vi "Keithley DMM6500 DAQ6500 Series Scanning Low Level DCV.vi"() -> ()   [LabVIEW 2016]
doc: "This example shows how to scan low level DC voltage."
uses:
  Public/Data/Read (Multiple Points).vi
  Keithley DMM6500 DAQ6500 Series.lvlib
panel:
  in  "Buffer Element2 ()":i32(ring) items=["", "Date", "Extra", "Formatted", "Fractional", "Reading", "Relative", "Seconds", "Status", "Time", "Tstamp", "Unit", "CHAN", "Extra Form", "Extra Unit"]
  in  "Buffer Element1 ()":i32(ring) items=["", "Date", "Extra", "Formatted", "Fractional", "Reading", "Relative", "Seconds", "Status", "Time", "Tstamp", "Unit", "CHAN", "Extra Format", "Extra Unit"]
  in  "File Name(\"/usb1/MyData.csv\")":string="/usb1/MyData.csv"
  out "Measurements":dbl[](array[numeric])
  in  "Scan Delay (0 s)":dbl
  in  "Power Line Cycle (1)":dbl=1.0
  in  "Scan Count (10)":u32=10
  in  "Buffer Size (10)":u32=10
  in  "Buffer Name(defbuffer1)":string="defbuffer1"
  in  "Channel List (\"101:106\")":string="101:106"
  in  "VISA resource name":refnum<visa-resource-name>
  # "(c) 2018 National Instruments.  ALL RIGHTS RESERVED."
  # "This example VI demonstrates how to use the DAQ6500 series to accurately measure DC voltage in a variety of ranges. To ensure accurate data, the NPLC (Number of Power Line Cycles) and autozero  options are used for this test."
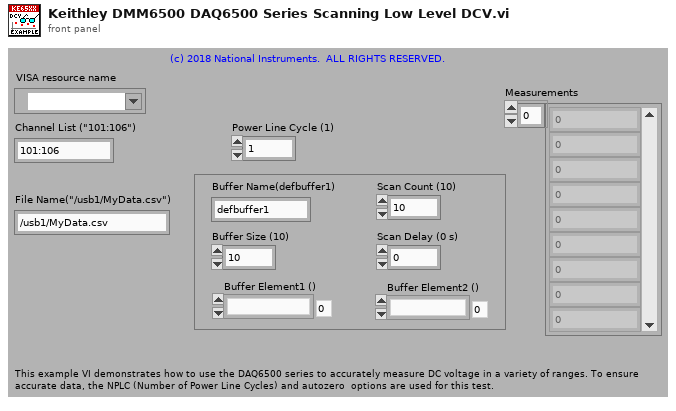
[diagram p1: front panel]
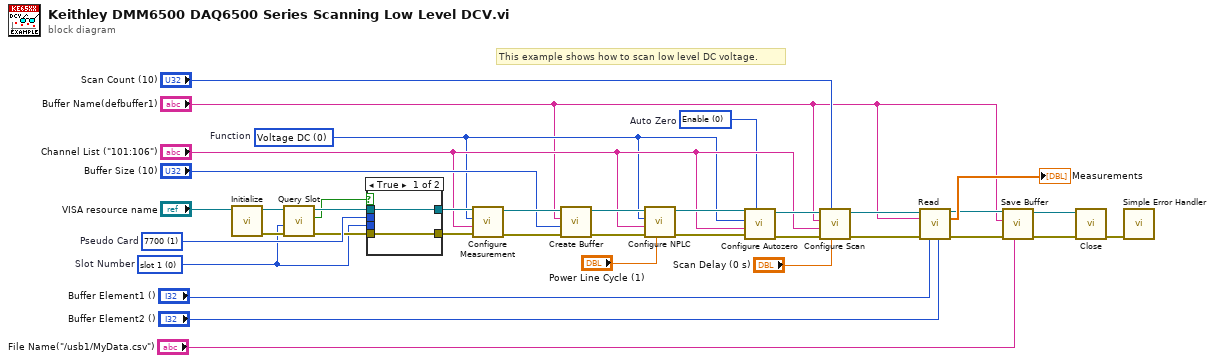
[diagram p0: block diagram]
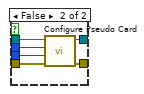
[diagram p2: hidden frame]
diagram:
  w4 = 0 items=["slot 1", "slot 2"]  # Slot Number
  w15 = 1 items=["0", "7700", "7701", "7702", "7703", "7705", "7706", "7707", "7708", "7709", "7710", "7711", "7712"]  # Pseudo Card
  w16 = u32 0 items=["Enable", "Disable", "Once"]  # Auto Zero
  w22 = 0 items=[" Voltage DC", "Voltage AC", "Current DC", "Current AC", "Resistance", "4-wire Resistance", "Diode", "Capacitance", "Temperature", "Continuity", "Frequency", "Period", "Voltage Ratio", "Digitize Voltage", "Digitize Current"]  # Function
  # "This example shows how to scan low level DC voltage."
  n1 = call "Initialize.vi"("VISA resource name"="VISA resource name") -> ("error out"=w7:errorcluster, "VISA resource name out"=w8:refnum<visa-resource-name>)  [unwired: 9 in]
  n2 = call "Query Slot.vi"("error in (no error)"=w7, "Slot Number(0: slot 1)"=w4, "VISA resource name"=w8) -> ("error out"=w6:errorcluster, "Real Card In Slot"=w3:bool, "VISA resource name out"=w5:refnum<visa-resource-name>)  [unwired: 6 in]
  n3 = case shown="True" w3 {
    tunnel: [w39 w45] -> w35
    tunnel: [w38 w44] -> w34
    tunnel: w15 -> [_ w43]
    tunnel: w6 -> [w38 w42]
    tunnel: w5 -> [w39 w41]
    tunnel: w4 -> [_ w40]
    frame True {
    }
    frame False {
      n4 = call "Configure Pseudo Card.vi"("error in (no error)"=w42, "Slot Number (0: slot1)"=w40, "Pseudo Card (0:No pseudocard)"=w43, "VISA resource name"=w41) -> ("error out"=w44:errorcluster, "VISA resource name out"=w45:refnum<visa-resource-name>)  [unwired: 6 in]
    }
  }
  n5 = call "Configure Measurement.vi"("error in (no error)"=w34, "Channel List(\"\")"="Channel List (\"101:106\")", "Function (0: Voltage DC)"=w22, "VISA resource name"=w35) -> ("error out"=w32:errorcluster, "VISA resource name out"=w33:refnum<visa-resource-name>)  [unwired: 6 in]
  n6 = call "Create Buffer.vi"("error in (no error)"=w32, "Buffer Size (10)"="Buffer Size (10)", "Buffer Name (\"\")"="Buffer Name(defbuffer1)", "VISA resource name"=w33) -> ("error out"=w29:errorcluster, "VISA resource name out"=w30:refnum<visa-resource-name>)  [unwired: 6 in]
  n7 = call "Configure NPLC.vi"("Power Line Cycle (1)"="Power Line Cycle (1)", "error in (no error)"=w29, "Channel List(\"\")"="Channel List (\"101:106\")", "Function (0: Voltage DC)"=w22, "VISA resource name"=w30) -> ("error out"=w27:errorcluster, "VISA resource name out"=w28:refnum<visa-resource-name>)  [unwired: 5 in]
  n8 = call "Configure Autozero.vi"("Auto Zero (0: Enable)"=w16, "error in (no error)"=w27, "Channel List(\"\")"="Channel List (\"101:106\")", "Function (0: Voltage DC)"=w22, "VISA resource name"=w28) -> ("error out"=w26:errorcluster, "VISA resource name out"=w25:refnum<visa-resource-name>)  [unwired: 5 in]
  n9 = call "Configure Scan.vi"("Delay Seconds (0 s)"="Scan Delay (0 s)", "Scan Count (1)"="Scan Count (10)", "error in (no error)"=w26, "Channel List(\"\")"="Channel List (\"101:106\")", "Reading Buffer (\"\")"="Buffer Name(defbuffer1)", "VISA resource name"=w25) -> ("error out"=w19:errorcluster, "VISA resource name out"=w20:refnum<visa-resource-name>)  [unwired: 4 in]
  n10 = call-poly "Read.vi"("VISA resource name"=w20, "Buffer Name (\"\")"="Buffer Name(defbuffer1)", "error in (no error)"=w19, "Buffer Element1 ()"="Buffer Element1 ()", "Buffer Element2 ()"="Buffer Element2 ()") -> ("VISA resource name out"=w13:refnum<visa-resource-name>, "Measurements"=→"Measurements":dbl[], "error out"=w12:errorcluster)  [unwired: 8 in]
  n11 = call "Save Buffer.vi"("File Name(\"\")"="File Name(\"/usb1/MyData.csv\")", "error in (no error)"=w12, "Buffer Name (\"\")"="Buffer Name(defbuffer1)", "VISA resource name"=w13) -> ("error out"=w11:errorcluster, "VISA resource name out"=w14:refnum<visa-resource-name>)  [unwired: 6 in]
  n12 = call "Close.vi"("error in (no error)"=w11, "VISA resource name"=w14) -> ("error out"=w37:errorcluster)  [unwired: 9 in]
  n13 = call <vilib>:"Simple Error Handler.vi"("error in (no error)"=w37) -> ()  [unwired: 4 in, 5 out]
